vi "Peristaltic_Pump.vi"(3 "Set state:":bool) -> (0 "Good Reply":bool, 2 "Comment":string)   [LabVIEW 2011]
uses:
  ADAM Client/Sub VIs/ADAM Controls/Address.ctl
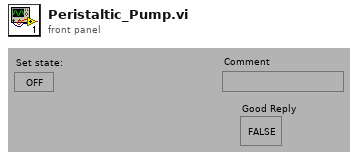
[diagram p1: front panel]
types:
  T1 = typedef "Address.ctl" = cluster{"Main":i32, "Ch.":i32, "Sub":i32, "Port Name":string}
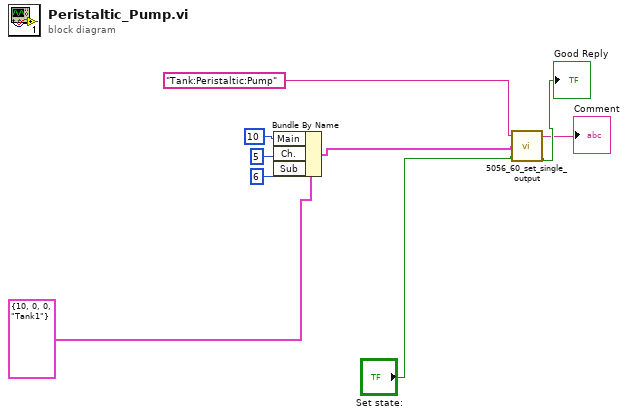
[diagram p0: block diagram]
diagram:
  n1 = Bundle By Name(cluster=T1 {"Main"=10, "Ch."=0, "Sub"=0, "Port Name"="Tank1"} ("Address (all reqd.)"), "Main"=10, "Ch."=5, "Sub"=6) -> (w4:T1)
  n2 = call "5056_60_set_single_output.vi"("Channel Name"="Tank:Peristaltic:Pump", "Address (all reqd.)"=w4, "Set state:"="Set state:") -> ("Comment"=→"Comment":string, "Good Reply"=→"Good Reply":bool)  [unwired: 2 in]
